vi "PS read config.vi"(2 "error in (no error)":errorcluster, 3 "Input Cluster":T1 {"MaxLambdaCurrent [A]" format="%.2f"; "LambdaRates [A/min]" format="%.5e"; "MaxNormalCurrent [A]" format="%.2f"; "StabilitySetting [%]" format="%.2f"; "FieldCurrentRatio [T/A]" format="%.2f"; "SwitchWaitTime [s]" format="%.2f"; "SwitchHtrCurrent [mA]" format="%.2f"; "TrainRates [A/min]" format="%.5e"; "NormalRates [A/min]" format="%.5e"; "Breakpts [A]" format="%.5e"}) -> (0 "error out":errorcluster, 1 "output cluster":T1 {"MaxLambdaCurrent [A]" format="%.2f"; "LambdaRates [A/min]" format="%.2f"; "MaxNormalCurrent [A]" format="%.2f"; "StabilitySetting [%]" format="%.2f"; "FieldCurrentRatio [T/A]" format="%.2f"; "SwitchWaitTime [s]" format="%.2f"; "SwitchHtrCurrent [mA]" format="%.2f"; "TrainRates [A/min]" format="%.2f"; "NormalRates [A/min]" format="%.2f"; "Breakpts [A]" format="%.2f"})   [LabVIEW 2019]
uses:
  <vilib>/Utility/error.llb/DialogType.ctl
  <vilib>/Utility/config.llb/Read Key (String).vi
  <vilib>/Utility/config.llb/NI_LVConfig.lvlib
panel:
  out "message":string=" INSTRUCTIONS:\r\rNormal Use:  When using subVIs that incorporate the error in/error out (or error I/O) structure, place this handler where you want to inform the user of an error, typically at the end of the I/O data path, as the last action of the program.  If the error in error? is ERROR, the handler creates a message describing the error and its source.  If the type of dialog = 1 (default), the message is displayed to the user, who can only acknowedge it.  If the type = 2, the user can acknowledge the message or abort execution; aborting a program with active I/O is not recommended.  If the type = 0, no message is displayed; this is used to process the error programmatically, and the error out cluster elements are wired to individual terminals for that reason.  \r\rOther Use:\n\r\nlocal testing.  To test the error code of a subVI or function that does not have the error I/O structure, you can wire its error code and a source string to the local error code and error source inputs.  If error in error? indicates no error and error code is not equal to 0, the local code and source are substituted for the error in values, and error? is set TRUE (ERROR)."
  out "key names":string[](array[string])
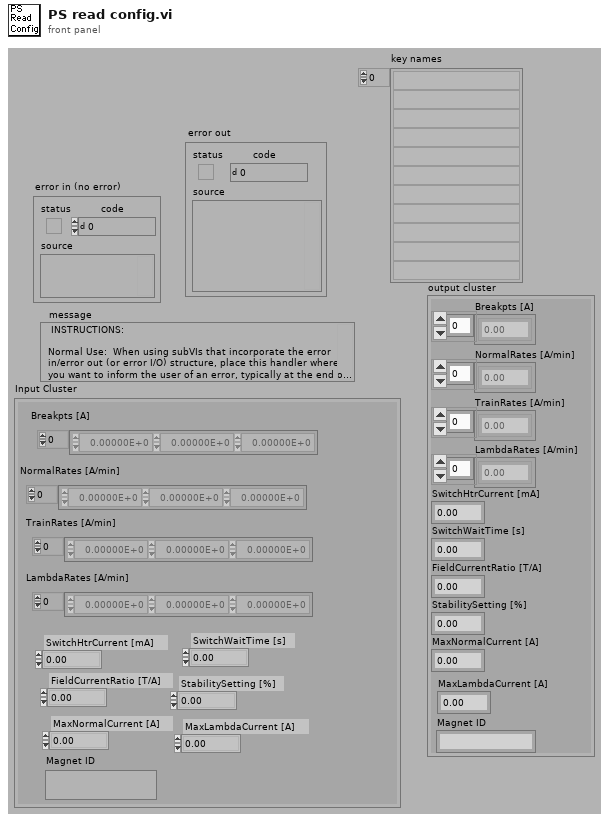
[diagram p1: front panel]
types:
  T1 = cluster{"Breakpts [A]":dbl[], "NormalRates [A/min]":dbl[], "TrainRates [A/min]":dbl[], "SwitchHtrCurrent [mA]":dbl, "SwitchWaitTime [s]":dbl, "FieldCurrentRatio [T/A]":dbl, "StabilitySetting [%]":dbl, "MaxNormalCurrent [A]":dbl, "Magnet ID":string, "LambdaRates [A/min]":dbl[], "MaxLambdaCurrent [A]":dbl}
  T2 = typedef "NI_LVConfig.lvlib/Config Data RefNum.ctl" = refnum<k1>
  T3 = typedef "DialogType.ctl" = u16
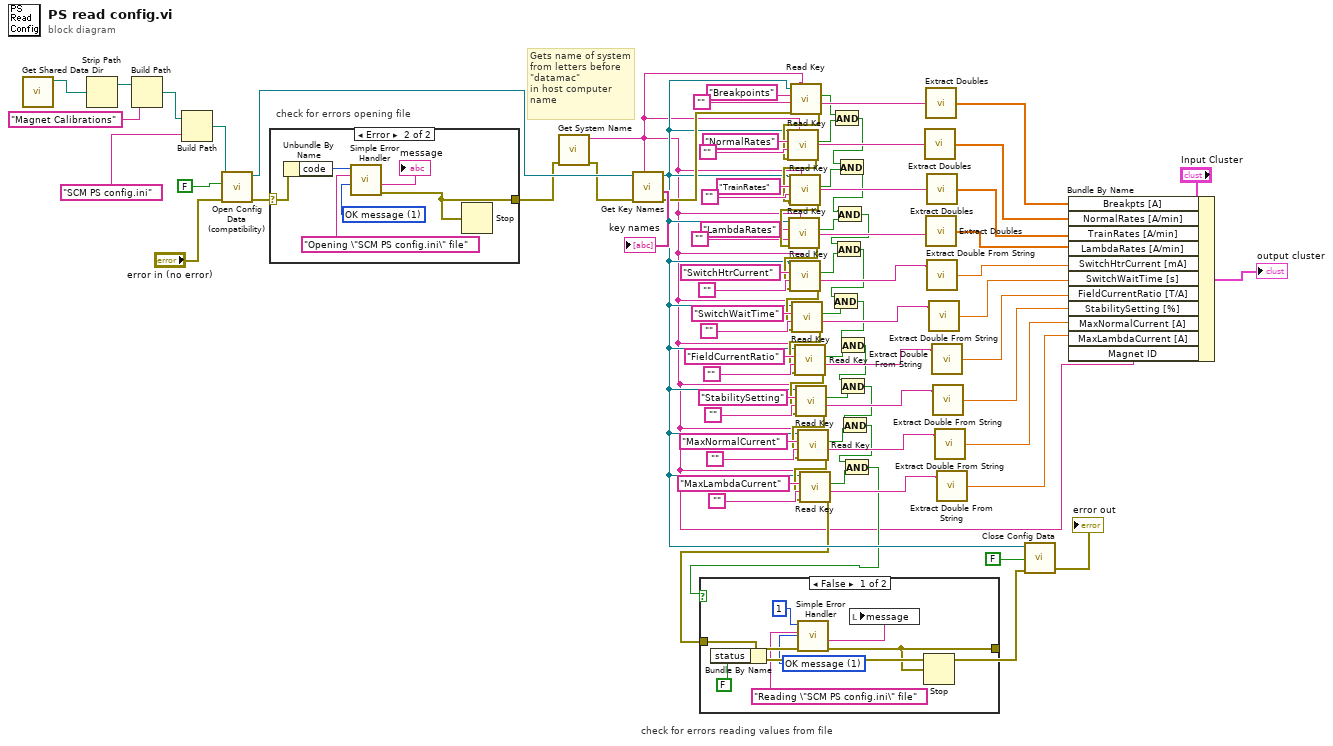
[diagram p0: block diagram]
diagram:
  # "Gets name of system\nfrom letters before \"datamac\" \nin host computer name"
  # "check for errors reading values from file"
  # "check for errors opening file"
  n1 = call "Get Shared Data Dir.vi"() -> ("Data Directory Path"=w6:path)  [unwired: 2 in, 1 out]
  n2 = Strip Path(path=w6) -> (stripped path=w5:path)  [unwired: 1 out]
  n3 = Build Path(base path=w5, name or relative path="Magnet Calibrations") -> (appended path=w3:path)
  n4 = Build Path(base path=w3, name or relative path="SCM PS config.ini") -> (appended path=w87:path)
  n5 = call <vilib>:"Open Config Data (compatibility).vi"("error in (no error)"="error in (no error)", "create file if necessary (T)"=FALSE ("create file if necessary? (T)"), "configuration file path"=w87) -> ("error out"=w8:errorcluster, "refnum"=w7:T2)  [unwired: 6 in, 1 out]
  n6 = case shown="Error" w8 {
    selector: w8 -> [w91 w93]
    tunnel: [w91 w95] -> w2
    frame No Error {
    }
    frame Error {
      w92 = T3 1 items=["no dialog", "OK message", "continue or stop message", "OK message + warnings", "continue/stop + warnings"] ("type of dialog (OK msg:1)")
      n7 = Unbundle By Name(w93) -> ("code"=w94:i32)
      n8 = call <vilib>:"Simple Error Handler.vi"("error code (no error:0)"=w94, "error source (\" \")"="Opening \"SCM PS config.ini\" file" ("error source (\" \")"), "type of dialog (OK msg:1)"=w92) -> ("source out"=→"message":string, "error out"=w95:errorcluster)  [unwired: 2 in, 3 out]
      n9 = Stop(stop? (T)=w95) -> ()
    }
  }
  n10 = call "Get System Name.vi"("error in (no error)"=w2) -> ("error out"=w1:errorcluster, "System Name"=w9:string)  [unwired: 5 in]
  n11 = call <vilib>:"Get Key Names.vi"("section"=w9, "error in (no error)"=w1, "refnum"=w7) -> ("error out"=w81:errorcluster, "key names"=→"key names":string[], "refnum out"=w16:T2)  [unwired: 5 in, 1 out]
  n12 = call-poly <vilib>:"Read Key.vi"("section"=w9, "error in (no error)"=w81, "default value"="", "key"="Breakpoints", "refnum"=w16) -> ("error out"=w78:errorcluster, "value"=w82:string, "found?"=w42:bool)  [unwired: 3 in, 1 out]
  n13 = call-poly <vilib>:"Read Key.vi"("section"=w9, "error in (no error)"=w78, "default value"="", "key"="NormalRates", "refnum"=w16) -> ("error out"=w73:errorcluster, "value"=w77:string, "found?"=w41:bool)  [unwired: 3 in, 1 out]
  n14 = call-poly <vilib>:"Read Key.vi"("section"=w9, "error in (no error)"=w73, "default value"="", "key"="TrainRates", "refnum"=w16) -> ("error out"=w29:errorcluster, "value"=w74:string, "found?"=w39:bool)  [unwired: 3 in, 1 out]
  n15 = call-poly <vilib>:"Read Key.vi"("section"=w9, "error in (no error)"=w29, "default value"="", "key"="LambdaRates", "refnum"=w16) -> ("error out"=w28:errorcluster, "value"=w23:string, "found?"=w25:bool)  [unwired: 3 in, 1 out]
  n16 = call-poly <vilib>:"Read Key.vi"("section"=w9, "error in (no error)"=w28, "default value"="", "key"="SwitchHtrCurrent", "refnum"=w16) -> ("error out"=w66:errorcluster, "value"=w70:string, "found?"=w38:bool)  [unwired: 3 in, 1 out]
  n17 = call-poly <vilib>:"Read Key.vi"("section"=w9, "error in (no error)"=w66, "default value"="", "key"="SwitchWaitTime", "refnum"=w16) -> ("error out"=w62:errorcluster, "value"=w67:string, "found?"=w36:bool)  [unwired: 3 in, 1 out]
  n18 = call-poly <vilib>:"Read Key.vi"("section"=w9, "error in (no error)"=w62, "default value"="", "key"="FieldCurrentRatio", "refnum"=w16) -> ("error out"=w58:errorcluster, "value"=w63:string, "found?"=w34:bool)  [unwired: 3 in, 1 out]
  n19 = call-poly <vilib>:"Read Key.vi"("section"=w9, "error in (no error)"=w58, "default value"="", "key"="StabilitySetting", "refnum"=w16) -> ("error out"=w54:errorcluster, "value"=w59:string, "found?"=w32:bool)  [unwired: 3 in, 1 out]
  n20 = call-poly <vilib>:"Read Key.vi"("section"=w9, "error in (no error)"=w54, "default value"="", "key"="MaxNormalCurrent", "refnum"=w16) -> ("error out"=w17:errorcluster, "value"=w55:string, "found?"=w30:bool)  [unwired: 3 in, 1 out]
  n21 = call-poly <vilib>:"Read Key.vi"("section"=w9, "error in (no error)"=w17, "default value"="", "key"="MaxLambdaCurrent", "refnum"=w16) -> ("error out"=w12:errorcluster, "value"=w19:string, "found?"=w18:bool)  [unwired: 3 in, 1 out]
  n22 = And(x=w42, y=w41) -> (x .and. y?=w40:bool)
  n23 = And(x=w40, y=w39) -> (x .and. y?=w26:bool)
  n24 = And(x=w26, y=w25) -> (x .and. y?=w11:bool)
  n25 = And(x=w11, y=w38) -> (x .and. y?=w37:bool)
  n26 = And(x=w37, y=w36) -> (x .and. y?=w35:bool)
  n27 = And(x=w35, y=w34) -> (x .and. y?=w33:bool)
  n28 = And(x=w33, y=w32) -> (x .and. y?=w31:bool)
  n29 = And(x=w31, y=w30) -> (x .and. y?=w14:bool)
  n30 = And(x=w14, y=w18) -> (x .and. y?=w13:bool)
  n31 = case shown="False" w13 {
    tunnel: [w99 w105] -> w53
    tunnel: w12 -> [w101 w105]
    frame False {
      w103 = u16 1 items=["no dialog", "OK message", "continue or stop message"] ("type of dialog (OK msg:1)")
      n32 = Bundle By Name(cluster=w101, "status"=FALSE) -> ()  [unwired: 1 out]
      n33 = call <vilib>:"Simple Error Handler.vi"("error code (no error:0)"=1, "error source (\" \")"="Reading \"SCM PS config.ini\" file" ("error source (\" \")"), "type of dialog (OK msg:1)"=w103) -> ("source out"=w102:string, "error out"=w99:errorcluster)  [unwired: 2 in, 3 out]
      n34 = local write "message"(w102) -> ()
      n35 = Stop(stop? (T)=w99) -> ()
    }
    frame True {
    }
  }
  n36 = call "Extract Doubles.vi"("String"=w77) -> ("Data"=w50:dbl[])  [unwired: 1 in]
  n37 = call "Extract Doubles.vi"("String"=w82) -> ("Data"=w52:dbl[])  [unwired: 1 in]
  n38 = call "Extract Doubles.vi"("String"=w23) -> ("Data"=w22:dbl[])  [unwired: 1 in]
  n39 = call "Extract Doubles.vi"("String"=w74) -> ("Data"=w49:dbl[])  [unwired: 1 in]
  n40 = call "Extract Double From String.vi"("string"=w70) -> ("floating pt. number"=w48:dbl)  [unwired: 1 in, 2 out]
  n41 = call "Extract Double From String.vi"("string"=w67) -> ("floating pt. number"=w47:dbl)  [unwired: 1 in, 2 out]
  n42 = call "Extract Double From String.vi"("string"=w63) -> ("floating pt. number"=w46:dbl)  [unwired: 1 in, 2 out]
  n43 = call "Extract Double From String.vi"("string"=w59) -> ("floating pt. number"=w45:dbl)  [unwired: 1 in, 2 out]
  n44 = call "Extract Double From String.vi"("string"=w55) -> ("floating pt. number"=w44:dbl)  [unwired: 1 in, 2 out]
  n45 = call "Extract Double From String.vi"("string"=w19) -> ("floating pt. number"=w15:dbl)  [unwired: 1 in, 2 out]
  n46 = call <vilib>:"Close Config Data.vi"("error in (no error)"=w53, "write file if changed (T)"=FALSE ("write configuration file? (T)"), "refnum"=w16) -> ("error out"=→"error out":errorcluster)  [unwired: 7 in, 1 out]
  n47 = Bundle By Name(cluster="Input Cluster", "Breakpts [A]"=w52, "NormalRates [A/min]"=w50, "TrainRates [A/min]"=w49, "LambdaRates [A/min]"=w22, "SwitchHtrCurrent [mA]"=w48, "SwitchWaitTime [s]"=w47, "FieldCurrentRatio [T/A]"=w46, "StabilitySetting [%]"=w45, "MaxNormalCurrent [A]"=w44, "MaxLambdaCurrent [A]"=w15, "Magnet ID"=w9) -> (→"output cluster":T1)
